vi "Teleop.vi"(10 "Match Info":T1={"Autonomous Elapsed Seconds"=0.0, "TeleOp Elapsed Seconds"=0.0, "Disabled Elapsed Seconds"=0.0, "Visited Autonomous"=FALSE, "Visited TeleOp"=FALSE, "Visited Disabled"=FALSE, "Autonomous Settings"={"Autonomous Style"=enum."Independent", "VI Refnum"=refnum}}, 11 "Call Context":T2) -> ()   [LabVIEW 2018]
doc: "This VI is called for each TeleOp packet received from the DS where the robot is not disabled. It is often used to read from the joysticks and update I/O or to update setpoints for timed control loops. It should complete and return within 20 milliseconds or it may miss DS packets."
uses:
  <vilib>/Rock Robotics/WPI/DriverStation/WPI_DriverStationDerivedRobotMode.ctl
  <vilib>/Rock Robotics/WPI/DriverStation/WPI_DriverStationMatch Info.ctl
  <vilib>/Rock Robotics/WPI/Solenoid/WPI_SolenoidValue.ctl
  <vilib>/Rock Robotics/WPI/Utilities/WPI_GetSetVariantRefNum.vi
  Robot Global Data.vi
  <vilib>/Rock Robotics/Network Tables/NT Write Numeric Array.vi
  <vilib>/Rock Robotics/WPI/Solenoid/WPI_SolenoidSetEnum.vi
  <vilib>/Rock Robotics/Network Tables/NT Write Number.vi
  <vilib>/Rock Robotics/Network Tables/NT Write Boolean Array.vi
  <vilib>/Rock Robotics/Network Tables/NT Read Boolean.vi
  <vilib>/Rock Robotics/Network Tables/NT Read Number.vi
panel:
  out "Sample Slider 0":dbl(slide) scale=0.0..5.0
  out "Sample Boolean 1":bool
  out "Sample Boolean 0":bool
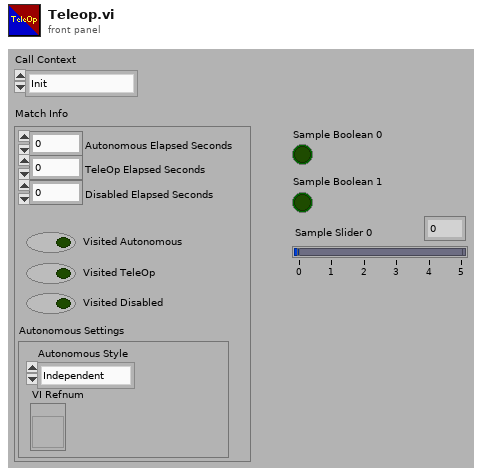
[diagram p1: front panel]
types:
  T1 = typedef "WPI_DriverStationMatch Info.ctl" = cluster{"Autonomous Elapsed Seconds":dbl, "TeleOp Elapsed Seconds":dbl, "Disabled Elapsed Seconds":dbl, "Visited Autonomous":bool, "Visited TeleOp":bool, "Visited Disabled":bool, "Autonomous Settings":cluster{"Autonomous Style":enum16{"Iterative", "Independent"}, "VI Refnum":refnum<vi>}}
  T2 = typedef "WPI_DriverStationDerivedRobotMode.ctl" = enum16{"Init", "Execute", "Stop"}
  T3 = typedef "WPI_SolenoidValue.ctl" = enum16{"Off", "On", "Forward", "Reverse"}
  T4 = typedef "WPI_JoystickDevRef.ctl" = cluster{"Device":T5}
  T5 = typedef "WPI_JoystickDeviceEnum.ctl" = enum16{"USB 0", "USB 1", "USB 2", "USB 3", "USB 4", "USB 5"}
  T6 = typedef "WPI_MotorControlDeviceRef.ctl" = cluster{"DeviceStatus":errorcluster, "Type":T7, "PWM":cluster{"PWM Channel":T8, "DeadBand":T9}, "CAN":cluster{"Device Number":u8, "SetOutput VI Ref":variant, "GetOutput VI Ref":variant, "Enable VI Ref":variant, "Disable VI Ref":variant, "Data":variant}, "Invert":bool, "DIO PWM":cluster{"PWM \"Enable\" Channel":T8, "DIOChannel":T10, "PWM Rate":dbl}}
  T7 = typedef "WPI_MotorControlType.ctl" = enum16{"PWM", "CAN", "DIO PWM"}
  T8 = typedef "FPGA_DIOPWMChannel.ctl" = enum8{"PWM 0", "PWM 1", "PWM 2", "PWM 3", "PWM 4", "PWM 5", "PWM 6", "PWM 7", "PWM 8", "PWM 9", "PWM MXP 0", "PWM MXP 1", "PWM MXP 2", "PWM MXP 3", "PWM MXP 4", "PWM MXP 5", "PWM MXP 6", "PWM MXP 7", "PWM MXP 8", "PWM MXP 9", "Invalid"}
  T9 = typedef "WPI_PWMDeadband.ctl" = cluster{"Name":string, "maxPositivePwm":i32, "minPositivePwm":i32, "centerPwm":i32, "maxNegativePwm":i32, "minNegativePwm":i32, "angularRange":u16}
  T10 = typedef "FPGA_DIOChannel.ctl" = enum8{"DIO 0", "DIO 1", "DIO 2", "DIO 3", "DIO 4", "DIO 5", "DIO 6", "DIO 7", "DIO 8", "DIO 9", "DIO MXP 0", "DIO MXP 1", "DIO MXP 2", "DIO MXP 3", "DIO MXP 4", "DIO MXP 5", "DIO MXP 6", "DIO MXP 7", "DIO MXP 8", "DIO MXP 9", "DIO MXP 10", "DIO MXP 11", "DIO MXP 12", "DIO MXP 13", "DIO MXP 14", "DIO MXP 15", "SPI Port CS1", "SPI Port CS2", "SPI Port CS3", "SPI Port MISO", "SPI Port MOSI", "Invalid"}
  T11 = typedef "WPI_RobotDriveDevRef.ctl" = cluster{"DevStatus":errorcluster, "Motors[]":T6[], "Square Inputs":bool, "Max Output":dbl}
  T12 = typedef "WPI_SolenoidDevRef.ctl" = cluster{"DevStatus":errorcluster, "Pneumatics Control Module":u8, "Forward Solenoid Channel":T13, "Reverse Solenoid Channel":T13}
  T13 = typedef "WPI_SolenoidChannel.ctl" = enum8{"Solenoid 0", "Solenoid 1", "Solenoid 2", "Solenoid 3", "Solenoid 4", "Solenoid 5", "Solenoid 6", "Solenoid 7", "Invalid"}
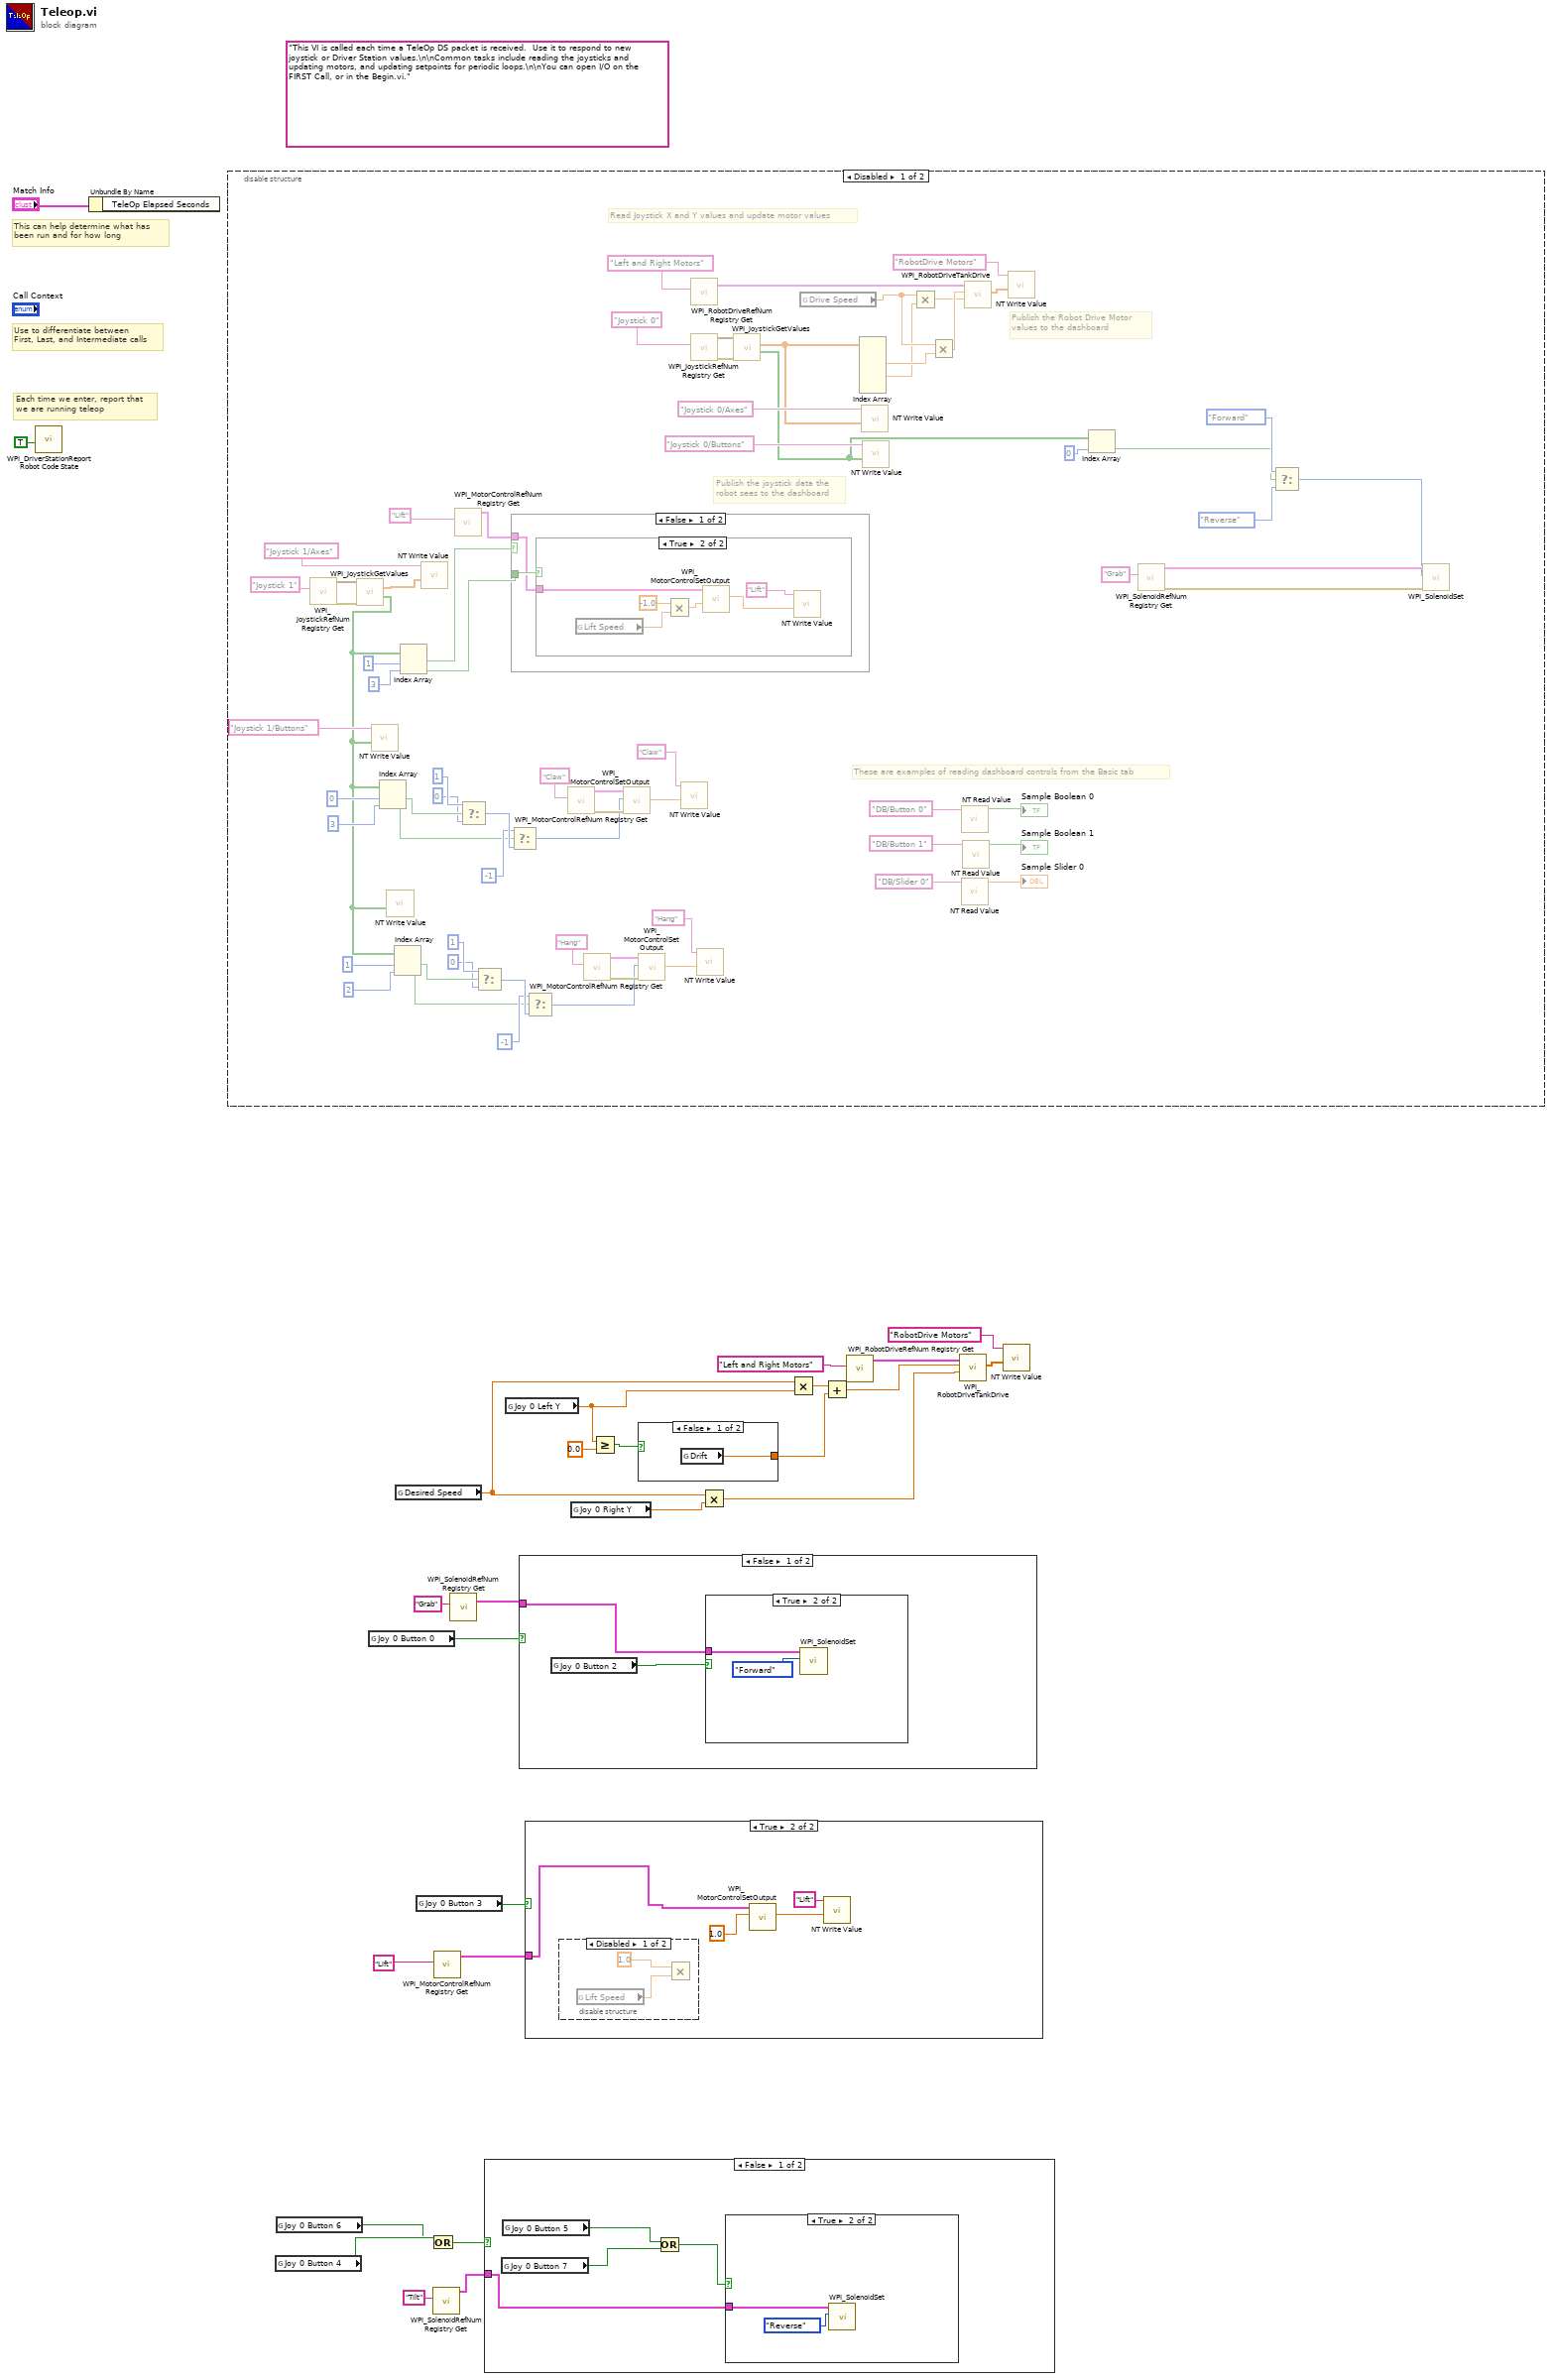
[diagram p0: block diagram]
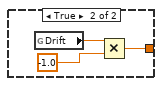
[diagram p2: hidden frame]
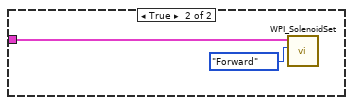
[diagram p4: hidden frame]
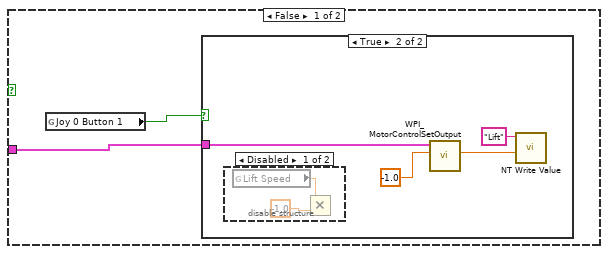
[diagram p5: hidden frame]
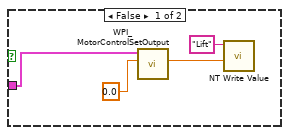
[diagram p6: hidden frame]
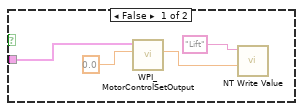
[diagram p9: hidden frame]
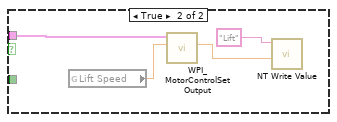
[diagram p10: hidden frame]
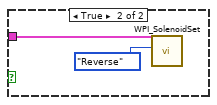
[diagram p13: hidden frame]
diagram:
  (unwired) "This VI is called each time a TeleOp DS packet is received.  Use it to respond to new joystick or Driver Station values.\n\nCommon tasks include reading the joysticks and updating motors, and updating setpoints for periodic loops.\n\nYou can open I/O on the FIRST Call, or in the Begin.vi."
  # "Each time we enter, report that\nwe are running teleop"
  # "Use to differentiate between\nFirst, Last, and Intermediate calls"
  # "This can help determine what has\nbeen run and for how long"
  n1 = call <vilib>:"WPI_DriverStationReport Robot Code State.vi"("TeleOp"=TRUE ("Autonomous")) -> ()  [unwired: 10 in, 1 out]
  n2 = Unbundle By Name("Match Info") -> ()  [unwired: 1 out]
  n3 = disable-structure shown="Disabled" {
    frame Disabled {
      # "These are examples of reading dashboard controls from the Basic tab"
      # "Publish the Robot Drive Motor\nvalues to the dashboard"
      # "Publish the joystick data the\nrobot sees to the dashboard"
      # "Read Joystick X and Y values and update motor values"
      n4 = call <vilib>:"WPI_JoystickRefNum Registry Get.vi"("refnum name"="Joystick 1") -> ("error out"=w78:errorcluster, "JoystickDevRef"=w83:T4)  [unwired: 9 in]
      n5 = call <vilib>:"WPI_JoystickGetValues.vi"("error in (no error)"=w78, "JoystickDevRef"=w83) -> ("Buttons"=w32:bool[], "Axes"=w79:dbl[])  [unwired: 5 in, 3 out]
      n6 = call-poly <vilib>:"NT Write Value.vi"("Boolean Array"=w32, "Name"="Joystick 1/Buttons") -> ()  [unwired: 9 in, 1 out]
      n7 = Index Array(array=w32, index #1=0, index #2=3) -> (element #1=w72:bool, element #2=w65:bool)
      n8 = call-poly <vilib>:"NT Write Value.vi"("Boolean Array"=w32) -> ()  [unwired: 10 in, 1 out]
      n9 = Index Array(array=w32, index #1=1, index #2=2) -> (element #1=w59:bool, element #2=w51:bool)
      n10 = Index Array(array=w32, index #1=1 ("index"), index #2=3 ("index")) -> (element #1=w29:bool, element #2=w27:bool)
      n11 = call-poly <vilib>:"NT Write Value.vi"("Numeric Array"=w79, "Name"="Joystick 1/Axes") -> ()  [unwired: 9 in, 1 out]
      n12 = call <vilib>:"WPI_MotorControlRefNum Registry Get.vi"("refnum name"="Lift") -> ("MotorControlDevRef"=w28:T6)  [unwired: 9 in, 1 out]
      n13 = Select(t=1, s=w72, f=0) -> (s? t:f=w67:i32)
      n14 = Select(t=1, s=w59, f=0) -> (s? t:f=w53:i32)
      n15 = case shown="False" w29 {
        tunnel: w28 -> [w98 w113]
        tunnel: w27 -> [w99 _]
        frame False {
          n16 = case shown="True" w99 {
            tunnel: w98 -> [w100 w107]
            frame False {
              n17 = call <vilib>:"WPI_MotorControlSetOutput.vi"("Output"=0.0, "MotorControlDevRef"=w100) -> ("Motor Output"=w102:dbl)  [unwired: 7 in, 2 out]
              n18 = call-poly <vilib>:"NT Write Value.vi"("Numeric"=w102, "Name"="Lift") -> ()  [unwired: 9 in, 1 out]
            }
            frame True {
              n19 = global read "Robot Global Data.vi" "Lift Speed"() -> (w105:dbl)
              n20 = Multiply(x=-1.0, y=w105) -> (x*y=w106:dbl)
              n21 = call <vilib>:"WPI_MotorControlSetOutput.vi"("options"=w106, "MotorControlDevRef"=w107) -> ("Motor Output"=w108:dbl)  [unwired: 7 in, 2 out]
              n22 = call-poly <vilib>:"NT Write Value.vi"("Numeric"=w108, "Name"="Lift") -> ()  [unwired: 9 in, 1 out]
            }
          }
        }
        frame True {
          n23 = global read "Robot Global Data.vi" "Lift Speed"() -> (w112:dbl)
          n24 = call <vilib>:"WPI_MotorControlSetOutput.vi"("Output"=w112, "MotorControlDevRef"=w113) -> ("Motor Output"=w110:dbl)  [unwired: 7 in, 2 out]
          n25 = call-poly <vilib>:"NT Write Value.vi"("Numeric"=w110, "Name"="Lift") -> ()  [unwired: 9 in, 1 out]
        }
      }
      n26 = Select(t=-1, s=w65, f=w67) -> (s? t:f=w37:i32)
      n27 = Select(t=-1, s=w51, f=w53) -> (s? t:f=w56:i32)
      n28 = call <vilib>:"WPI_MotorControlRefNum Registry Get.vi"("refnum name"="Claw") -> ("error out"=w74:errorcluster, "MotorControlDevRef"=w75:T6)  [unwired: 9 in]
      n29 = call <vilib>:"WPI_MotorControlRefNum Registry Get.vi"("refnum name"="Hang") -> ("error out"=w61:errorcluster, "MotorControlDevRef"=w62:T6)  [unwired: 9 in]
      n30 = call <vilib>:"WPI_MotorControlSetOutput.vi"("error in (no error)"=w74, "Output"=w37, "MotorControlDevRef"=w75) -> ("Motor Output"=w64:dbl)  [unwired: 6 in, 2 out]
      n31 = call <vilib>:"WPI_MotorControlSetOutput.vi"("error in (no error)"=w61, "Output"=w56, "MotorControlDevRef"=w62) -> ("Motor Output"=w50:dbl)  [unwired: 6 in, 2 out]
      n32 = call-poly <vilib>:"NT Write Value.vi"("Numeric"=w64, "Name"="Claw") -> ()  [unwired: 9 in, 1 out]
      n33 = call <vilib>:"WPI_RobotDriveRefNum Registry Get.vi"("refnum name"="Left and Right Motors") -> ("RobotDriveDevRef"=w76:T11)  [unwired: 1 in, 9 out]
      n34 = call <vilib>:"WPI_JoystickRefNum Registry Get.vi"("refnum name"="Joystick 0") -> ("error out"=w41:errorcluster, "JoystickDevRef"=w95:T4)  [unwired: 1 in, 8 out]
      n35 = call-poly <vilib>:"NT Write Value.vi"("Numeric"=w50, "Name"="Hang") -> ()  [unwired: 9 in, 1 out]
      n36 = call <vilib>:"WPI_JoystickGetValues.vi"("error in (no error)"=w41, "JoystickDevRef"=w95) -> ("Buttons"=w42:bool[], "Axes"=w92:dbl[])  [unwired: 5 in, 3 out]
      n37 = global read "Robot Global Data.vi" "Drive Speed"() -> (w34:dbl)
      n38 = Index Array(array=w92) -> (element #2=w48:dbl, element #4=w33:dbl)  [unwired: 6 in, 4 out]
      n39 = call-poly <vilib>:"NT Write Value.vi"("Numeric Array"=w92, "Name"="Joystick 0/Axes") -> ()  [unwired: 9 in, 1 out]
      n40 = call-poly <vilib>:"NT Write Value.vi"("Boolean Array"=w42, "Name"="Joystick 0/Buttons") -> ()  [unwired: 9 in, 1 out]
      n41 = Multiply(x=w34, y=w33) -> (x*y=w35:dbl)
      n42 = Multiply(x=w34, y=w48) -> (x*y=w47:dbl)
      n43 = call-poly <vilib>:"NT Read Value.vi"("Name"="DB/Button 0" ("refnum name")) -> ("Boolean"=→"Sample Boolean 0":bool)  [unwired: 9 in, 1 out]
      n44 = call-poly <vilib>:"NT Read Value.vi"("Name"="DB/Slider 0" ("refnum name")) -> ("Numeric"=→"Sample Slider 0":dbl)  [unwired: 9 in, 1 out]
      n45 = call-poly <vilib>:"NT Read Value.vi"("Name"="DB/Button 1" ("refnum name")) -> ("Boolean"=→"Sample Boolean 1":bool)  [unwired: 9 in, 1 out]
      n46 = call <vilib>:"WPI_RobotDriveTankDrive.vi"("Right axis value"=w35, "Left axis value"=w47, "RobotDriveDevRef"=w76) -> ("Motor Values"=w77:dbl[])  [unwired: 6 in, 2 out]
      n47 = call-poly <vilib>:"NT Write Value.vi"("Numeric Array"=w77, "Name"="RobotDrive Motors") -> ()  [unwired: 9 in, 1 out]
      n48 = Index Array(array=w42, index=0) -> (element=w38:bool)
      n49 = call <vilib>:"WPI_SolenoidRefNum Registry Get.vi"("refnum name"="Grab") -> ("error out"=w43:errorcluster, "SolenoidDevRef"=w44:T12)  [unwired: 9 in]
      n50 = Select(t=WPI_SolenoidValue."Forward" ("Value"), s=w38, f=WPI_SolenoidValue."Reverse" ("Value")) -> (s? t:f=w36:T3)
      n51 = call-poly <vilib>:"WPI_SolenoidSet.vi"("error in (no error)"=w43, "Value"=w36, "SolenoidDevRef"=w44) -> ()  [unwired: 7 in, 2 out]
    }
    frame Enabled {
    }
  }
  n52 = global read "Robot Global Data.vi" "Joy 0 Button 4"() -> (w9:bool)
  n53 = global read "Robot Global Data.vi" "Joy 0 Button 6"() -> (w8:bool)
  n54 = global read "Robot Global Data.vi" "Joy 0 Button 0"() -> (w13:bool)
  n55 = global read "Robot Global Data.vi" "Desired Speed"() -> (w24:dbl)
  n56 = global read "Robot Global Data.vi" "Joy 0 Button 3"() -> (w11:bool)
  n57 = Or(x=w8, y=w9) -> (x .or. y?=w7:bool)
  n58 = call <vilib>:"WPI_SolenoidRefNum Registry Get.vi"("refnum name"="Tilt") -> ("SolenoidDevRef"=w5:T12)  [unwired: 9 in, 1 out]
  n59 = call <vilib>:"WPI_MotorControlRefNum Registry Get.vi"("refnum name"="Lift") -> ("MotorControlDevRef"=w10:T6)  [unwired: 9 in, 1 out]
  n60 = call <vilib>:"WPI_SolenoidRefNum Registry Get.vi"("refnum name"="Grab") -> ("SolenoidDevRef"=w14:T12)  [unwired: 9 in, 1 out]
  n61 = case shown="False" w7 {
    tunnel: w5 -> [w114 w120]
    frame False {
      n62 = global read "Robot Global Data.vi" "Joy 0 Button 7"() -> (w117:bool)
      n63 = global read "Robot Global Data.vi" "Joy 0 Button 5"() -> (w116:bool)
      n64 = Or(x=w116, y=w117) -> (x .or. y?=w115:bool)
      n65 = case shown="True" w115 {
        tunnel: w114 -> [_ w118]
        frame False {
        }
        frame True {
          n66 = call-poly <vilib>:"WPI_SolenoidSet.vi"("Value"=WPI_SolenoidValue."Reverse", "SolenoidDevRef"=w118) -> ()  [unwired: 8 in, 2 out]
        }
      }
    }
    frame True {
      n67 = call-poly <vilib>:"WPI_SolenoidSet.vi"("Value"=WPI_SolenoidValue."Forward", "SolenoidDevRef"=w120) -> ()  [unwired: 8 in, 2 out]
    }
  }
  n68 = global read "Robot Global Data.vi" "Joy 0 Left Y"() -> (w3:dbl)
  n69 = case shown="False" w13 {
    tunnel: w14 -> [w122 w127]
    frame False {
      n70 = global read "Robot Global Data.vi" "Joy 0 Button 2"() -> (w123:bool)
      n71 = case shown="True" w123 {
        tunnel: w122 -> [_ w124]
        frame False {
        }
        frame True {
          n72 = call-poly <vilib>:"WPI_SolenoidSet.vi"("Value"=WPI_SolenoidValue."Forward", "SolenoidDevRef"=w124) -> ()  [unwired: 8 in, 2 out]
        }
      }
    }
    frame True {
      n73 = call-poly <vilib>:"WPI_SolenoidSet.vi"("Value"=WPI_SolenoidValue."Reverse", "SolenoidDevRef"=w127) -> ()  [unwired: 8 in, 2 out]
    }
  }
  n74 = case shown="True" w11 {
    tunnel: w10 -> [w128 w141]
    frame False {
      n75 = global read "Robot Global Data.vi" "Joy 0 Button 1"() -> (w129:bool)
      n76 = case shown="True" w129 {
        tunnel: w128 -> [w130 w135]
        frame False {
          n77 = call <vilib>:"WPI_MotorControlSetOutput.vi"("Output"=0.0, "MotorControlDevRef"=w130) -> ("Motor Output"=w132:dbl)  [unwired: 7 in, 2 out]
          n78 = call-poly <vilib>:"NT Write Value.vi"("Numeric"=w132, "Name"="Lift") -> ()  [unwired: 9 in, 1 out]
        }
        frame True {
          n79 = disable-structure shown="Disabled" {
            frame Disabled {
              n80 = global read "Robot Global Data.vi" "Lift Speed"() -> (w139:dbl)
              n81 = Multiply(x=w139, y=-1.0) -> ()  [unwired: 1 out]
            }
            frame Enabled {
            }
          }
          n82 = call <vilib>:"WPI_MotorControlSetOutput.vi"("Output"=-1.0, "MotorControlDevRef"=w135) -> ("Motor Output"=w136:dbl)  [unwired: 7 in, 2 out]
          n83 = call-poly <vilib>:"NT Write Value.vi"("Numeric"=w136, "Name"="Lift") -> ()  [unwired: 9 in, 1 out]
        }
      }
    }
    frame True {
      n84 = disable-structure shown="Disabled" {
        frame Disabled {
          n85 = global read "Robot Global Data.vi" "Lift Speed"() -> (w145:dbl)
          n86 = Multiply(x=1.0, y=w145) -> ()  [unwired: 1 out]
        }
        frame Enabled {
        }
      }
      n87 = call <vilib>:"WPI_MotorControlSetOutput.vi"("Output"=1.0, "MotorControlDevRef"=w141) -> ("Motor Output"=w142:dbl)  [unwired: 7 in, 2 out]
      n88 = call-poly <vilib>:"NT Write Value.vi"("Numeric"=w142, "Name"="Lift") -> ()  [unwired: 9 in, 1 out]
    }
  }
  n89 = global read "Robot Global Data.vi" "Joy 0 Right Y"() -> (w23:dbl)
  n90 = Greater Or Equal?(x=w3, y=0.0) -> (x >= y?=w4:bool)
  n91 = case shown="False" w4 {
    tunnel: [w146 w147] -> w1
    frame False {
      n92 = global read "Robot Global Data.vi" "Drift"() -> (w146:dbl)
    }
    frame True {
      n93 = global read "Robot Global Data.vi" "Drift"() -> (w149:dbl)
      n94 = Multiply(x=w149, y=-1.0) -> (x*y=w147:dbl)
    }
  }
  n95 = Multiply(x=w24, y=w23) -> (x*y=w16:dbl)
  n96 = Multiply(x=w24, y=w3) -> (x*y=w22:dbl)
  n97 = Add(x=w22, y=w1) -> (x+y=w17:dbl)
  n98 = call <vilib>:"WPI_RobotDriveRefNum Registry Get.vi"("refnum name"="Left and Right Motors") -> ("RobotDriveDevRef"=w18:T11)  [unwired: 1 in, 9 out]
  n99 = call <vilib>:"WPI_RobotDriveTankDrive.vi"("Right axis value"=w16, "Left axis value"=w17, "RobotDriveDevRef"=w18) -> ("Motor Values"=w19:dbl[])  [unwired: 6 in, 2 out]
  n100 = call-poly <vilib>:"NT Write Value.vi"("Numeric Array"=w19, "Name"="RobotDrive Motors") -> ()  [unwired: 9 in, 1 out]
